vi "hmi_shutdown.vi"(7 "hmi_references":T1, 8 "error in (no error)":errorcluster) -> (0 "error out":errorcluster)   [LabVIEW 2015, in "lv-interface-sub-re.lvlib"]
uses:
  lv-interface-sub-re.lvlib
  _controls/hmi_references.ctl
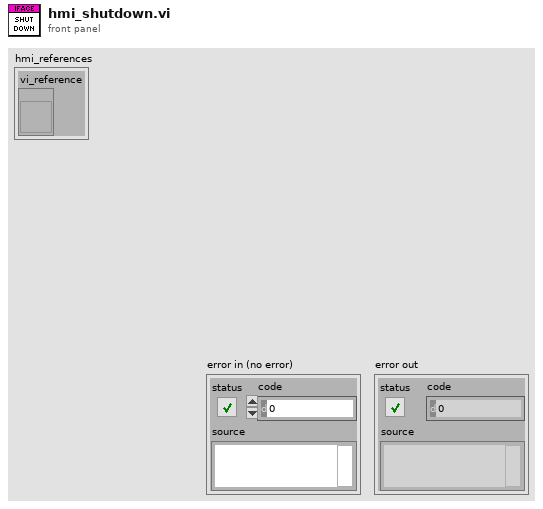
[diagram p1: front panel]
types:
  T1 = typedef "lv-interface-sub-re.lvlib/hmi_references.ctl" = cluster{"vi_reference":refnum<vi>}
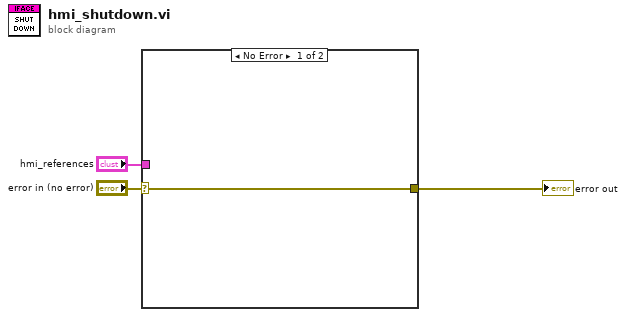
[diagram p0: block diagram]
diagram:
  n1 = case shown="No Error" "error in (no error)" {
    selector: "error in (no error)" -> [w4 w5]
    tunnel: [w4 w5] -> w2
    tunnel: "hmi_references" -> [_ _]
    frame No Error {
    }
    frame Error {
    }
  }
  "error out" <- w2
